vi "Rio_Pickup_Kicker (DONE).vi"(8 "error in (no error)":errorcluster) -> (0 "error out":errorcluster)   [LabVIEW 2017]
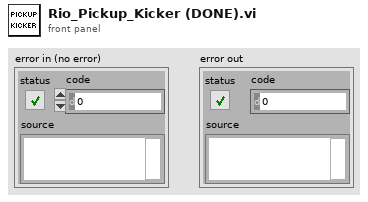
[diagram p1: front panel]
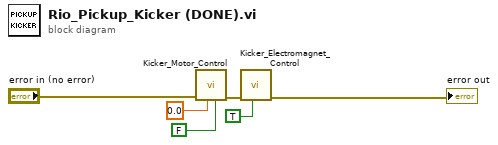
[diagram p0: block diagram]
diagram:
  n1 = call "Kicker_Motor_Control.vi"("Motor Dir (T/F = U/D)"=FALSE ("Motor Dir"), "Duty Cycle"=0.0 ("Motor Speed"), "error in"="error in (no error)") -> ("error out"=w1:errorcluster)  [unwired: 8 in]
  n2 = call "Kicker_Electromagnet_Control.vi"("Mag Enable"=TRUE, "error in"=w1) -> ("error out"=→"error out":errorcluster)  [unwired: 9 in]
